vi "Insert Error.vi"(8 "Message":string, 9 "Insert (T)":bool=TRUE, 10 "Code (5000)":i32=5000, 11 "Error In":errorcluster) -> (3 "Error Out":errorcluster)   [LabVIEW 2014, in "Endigit.lvlib"]
uses:
  Endigit.lvlib
panel:
  # "NOTICE - YOU MUST NOT REMOVE THIS NOTICE. PER THE FOLLOWING LICENSE, YOU MAY REPRODUCE THIS SOFTWARE PROVIDED YOU FOLLOW THE TERMS\nOF THE LICENSE.\n\n---BEGIN BSD LICENSE (http://opensource.org/licenses/BSD-2-Clause)---\nCopyright (c) 2015, Endigit, Inc. <robert@endigit.com>\nAll rights reserved.\n\nRedistribution and use in source and binary forms, with or without modification, are permitted provided that the following conditions are met:\n\n1. Redistributions of source code must retain the above copyright notice, this list of conditions and the following disclaimer.\n\n2. Redistributions in binary form must reproduce the above copyright notice, this list of conditions and the following disclaimer in the documentation and/or other \nmaterials provided with the distribution.\n\nTHIS SOFTWARE IS PROVIDED BY THE COPYRIGHT HOLDERS AND CONTRIBUTORS \"AS IS\" AND ANY EXPRESS OR IMPLIED WARRANTIES, INCLUDING, BUT NOT \nLIMITED TO, THE IMPLIED WARRANTIES OF MERCHANTABILITY AND FITNESS FOR A PARTICULAR PURPOSE ARE DISCLAIMED. IN NO EVENT SHALL THE COPYRIGHT \nHOLDER OR CONTRIBUTORS BE LIABLE FOR ANY DIRECT, INDIRECT, INCIDENTAL, SPECIAL, EXEMPLARY, OR CONSEQUENTIAL DAMAGES (INCLUDING, BUT NOT \nLIMITED TO, PROCUREMENT OF SUBSTITUTE GOODS OR SERVICES; LOSS OF USE, DATA, OR PROFITS; OR BUSINESS INTERRUPTION) HOWEVER CAUSED AND ON \nANY THEORY OF LIABILITY, WHETHER IN CONTRACT, STRICT LIABILITY, OR TORT (INCLUDING NEGLIGENCE OR OTHERWISE) ARISING IN ANY WAY OUT OF THE USE \nOF THIS SOFTWARE, EVEN IF ADVISED OF THE POSSIBILITY OF SUCH DAMAGE.\n---END BSD LICENSE---"
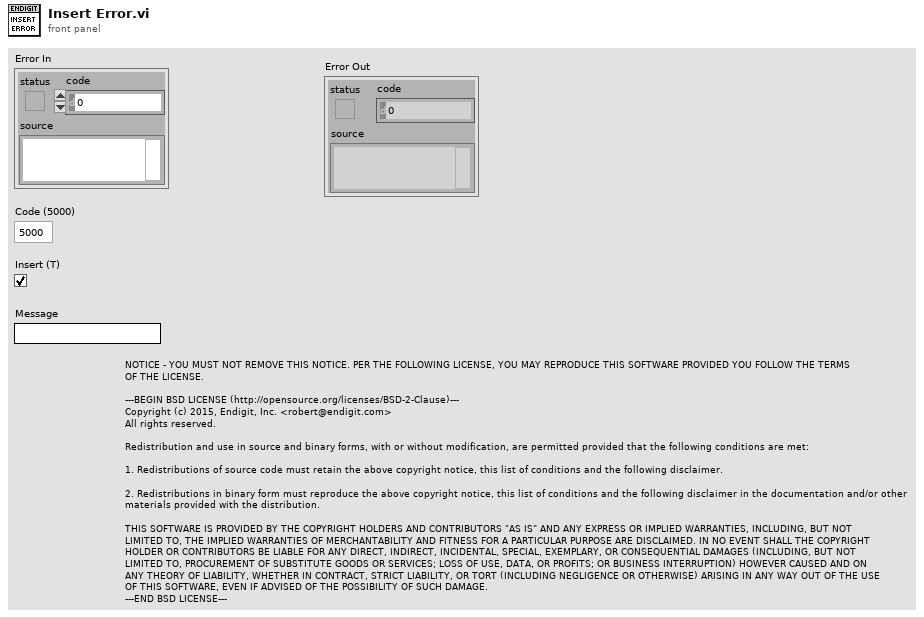
[diagram p1: front panel]
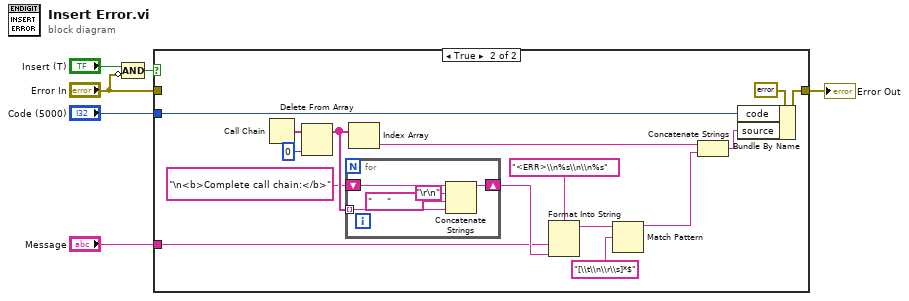
[diagram p0: block diagram]
diagram:
  n1 = Compound Arithmetic op=AND("Insert (T)", invert "Error In") -> (w1:bool)
  n2 = case shown="True" w1 {
    tunnel: [w7 w22] -> w2
    tunnel: "Code (5000)" -> [_ w8]
    tunnel: "Error In" -> [w7 _]
    tunnel: "Message" -> [_ w16]
    frame False {
    }
    frame True {
      n3 = Call Chain() -> (call chain=w19:string[])
      n4 = Delete From Array(array=w19, index=0) -> (array with subset deleted=w11:string[])  [unwired: 1 in, 1 out]
      n5 = for {
        tunnel: w11 -> [w24] mode=indexing
        shift-right: [w27] -> w17
        shift-left: "\n<b>Complete call chain:</b>" ("call chain header") -> [w25]
        n6 = Concatenate Strings(w25, "\r\n", "     ", w24) -> (w27:string)
      }
      n7 = Index Array(array=w11) -> (element=w13:string)  [unwired: 1 in]
      n8 = Format Into String(format string="<ERR>\\n%s\\n\\n%s", w16, w17) -> (resulting string=w14:string)  [unwired: 2 in, 1 out]
      n9 = Match Pattern(string=w14, regular expression="[\\t\\n\\r\\s]*$") -> (before substring=w9:string)  [unwired: 1 in, 3 out]
      n10 = Concatenate Strings(w13, w9) -> (w20:string)
      n11 = Bundle By Name(cluster=errorcluster {"status"=TRUE, "code"=0, "source"=""} ("error out"), "code"=w8, "source"=w20) -> (w22:errorcluster)
    }
  }
  "Error Out" <- w2
